vi "even elements.vi"(11 "Numeric":i32) -> (3 "Even? (count of program)":bool)   [LabVIEW 2015]
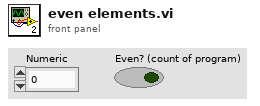
[diagram p1: front panel]
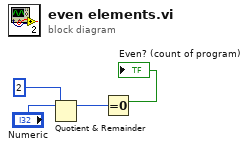
[diagram p0: block diagram]
diagram:
  n1 = Quotient & Remainder(x="Numeric", y=2) -> (x-y*floor(x/y)=w2:i32)  [unwired: 1 out]
  n2 = Equal To 0?(x=w2) -> (x = 0?=→"Even? (count of program)":bool)
